vi "max and min.vi"() -> ()   [LabVIEW 2012]
panel:
  in  "Tab Control":T1(tab)
  in  "Numeric":dbl
  in  "Numeric 2":dbl
  out "max(x,y)":dbl
  out "min(x,y)":dbl
  in  "Array":dbl[][](array[numeric])
  out "max value":dbl
  out "min value":dbl
  in  "String":string
  in  "String 2":string
  out "max(x,y) 2":string
  out "min(x,y) 2":string
  in  "Cluster":cluster{"String":string, "Numeric":dbl}
  in  "Cluster 2":cluster{"String":string, "Numeric":dbl}
  out "max(x,y) 3":cluster{"String":string, "Numeric":dbl}
  out "min(x,y) 3":cluster{"String":string, "Numeric":dbl}
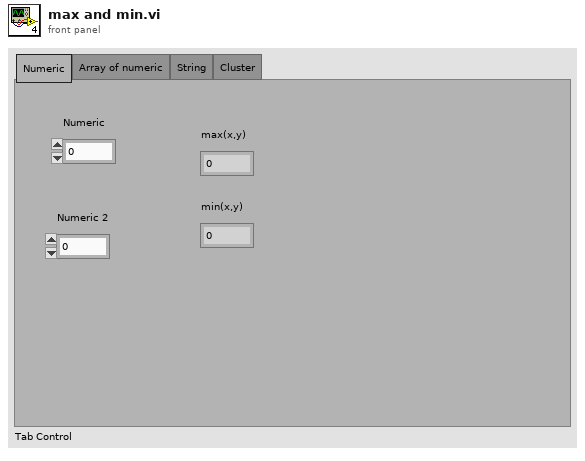
[diagram p1: front panel]
types:
  T1 = enum32{"Numeric", "Array of numeric", "String", "Cluster"}
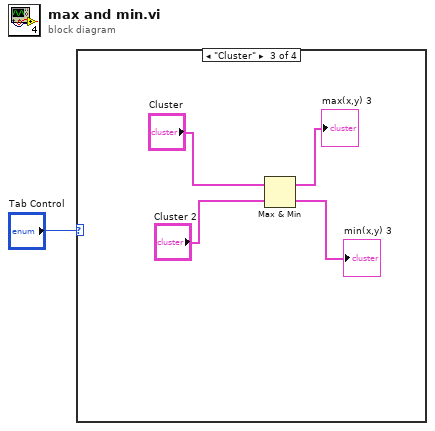
[diagram p0: block diagram]
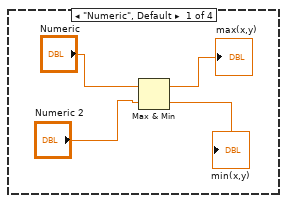
[diagram p2: hidden frame]
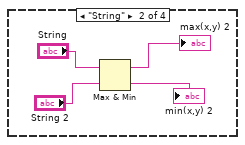
[diagram p3: hidden frame]
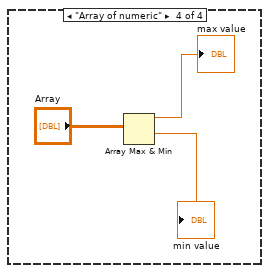
[diagram p4: hidden frame]
diagram:
  n1 = case shown="\"Cluster\"" "Tab Control" {
    frame "Numeric", Default {
      n2 = Max & Min(x="Numeric", y="Numeric 2") -> (max(x,y)=→"max(x,y)":dbl, min(x,y)=→"min(x,y)":dbl)
    }
    frame "String" {
      n3 = Max & Min(x="String", y="String 2") -> (max(x,y)=→"max(x,y) 2":string, min(x,y)=→"min(x,y) 2":string)
    }
    frame "Cluster" {
      n4 = Max & Min(x="Cluster", y="Cluster 2") -> (max(x,y)=→"max(x,y) 3":cluster{"String":string, "Numeric":dbl}, min(x,y)=→"min(x,y) 3":cluster{"String":string, "Numeric":dbl})
    }
    frame "Array of numeric" {
      n5 = Array Max & Min(array="Array") -> (max value=→"max value":dbl, min value=→"min value":dbl)  [unwired: 2 out]
    }
  }
